vi "SR Instruction.vi"(4 "Reset":bool, 5 "Set":bool) -> (1 "Status":bool)   [LabVIEW 2019]
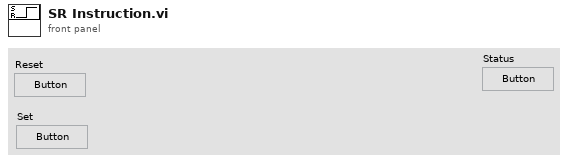
[diagram p1: front panel]
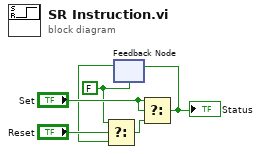
[diagram p0: block diagram]
diagram:
  w1 = FALSE
  n1 = feedback #1(w1) -> (w3:bool)
  n2 = Select(t=w1, s="Reset", f=w3) -> (s? t:f=w5:bool)
  n3 = Select(t="Set", s="Set", f=w5) -> (s? t:f=w2:bool)
  "Status" <- w2
  n4 = feedback-in #1(w2) -> ()
